vi "prueba_guardado_tags.vi"   [LabVIEW 2015]
uses:
  <vilib>/Utility/file.llb/Write Delimited Spreadsheet (string).vi
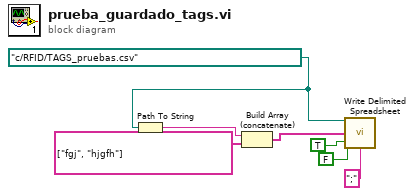
[diagram p0: block diagram]
diagram:
  w3 = path "c:/RFID/TAGS_pruebas.csv" ("file path (use dialog)")
  n1 = Path To String(path=w3) -> (string=w4:string)
  n2 = Build Array (concatenate)(w4, string[] ["fgj", "hjgfh"] ("array")) -> (w1:string[])
  n3 = call-poly <vilib>:"Write Delimited Spreadsheet.vi"("file path (dialog if empty)"=w3, "1D data"=w1, "append to file? (F)"=FALSE ("transpose? (no:F)"), "transpose? (F)"=TRUE ("append to file? (new file:F)"), "delimiter (\\t)"=";" ("delimiter (\\t)")) -> ()  [unwired: 9 in, 2 out]
